vi "Boolean Array to Matlab String.vi"(8 "error in (no error)":errorcluster, 10 "Value":bool[][](array[boolean]), 11 "Variable name":string) -> (0 "error out":errorcluster, 3 "String":string)   [LabVIEW 2014, in "Matlab API.lvlib"]
uses:
  Matlab API.lvlib
panel:
  out "Array":u8[](array[numeric]) format="%x"
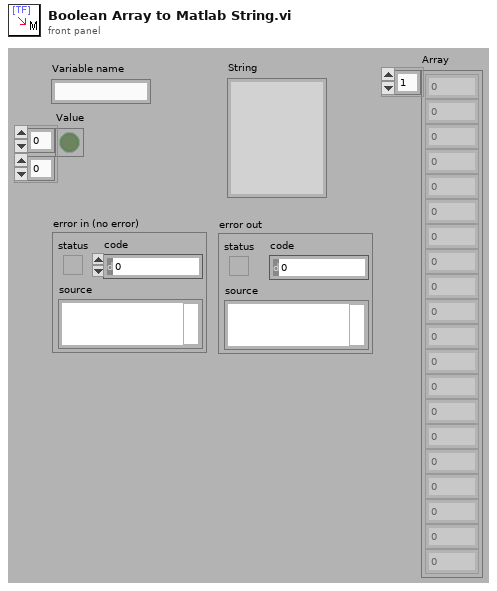
[diagram p1: front panel]
types:
  T1 = enum16{"big-endian, network order", "native, host order", "little-endian"}
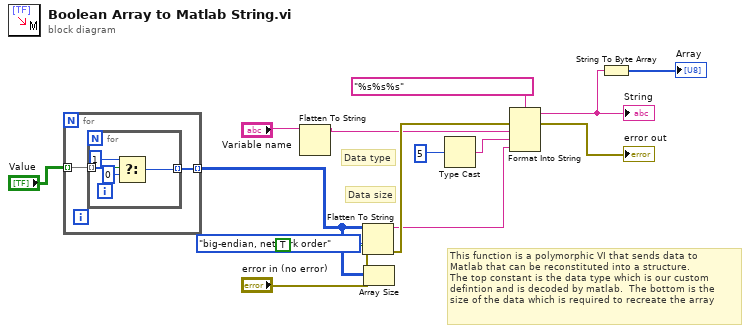
[diagram p0: block diagram]
diagram:
  # "Data size"
  # "Data type"
  # "This function is a polymorphic VI that sends data to\nMatlab that can be reconstituted into a structure.\nThe top constant is the data type which is our custom\ndefintion and is decoded by matlab.  The bottom is the\nsize of the data which is required to recreate the array"
  n1 = for {
    tunnel: "Value" -> [w17] mode=indexing
    tunnel: [w16] -> w1 mode=indexing
    n2 = for {
      tunnel: w17 -> [w21] mode=indexing
      tunnel: [w20] -> w16 mode=indexing
      n3 = Select(t=u8 1, s=w21, f=u8 0) -> (s? t:f=w20:u8)
    }
  }
  n4 = Flatten To String(anything="Variable name") -> (data string=w6:string)  [unwired: 1 in, 4 out]
  n5 = Flatten To String(anything=w1, prepend array or string size? (T)=TRUE, byte order (0:big-endian, network order)=T1."big-endian, network order", error in (no error)="error in (no error)") -> (data string=w3:string, error out=w12:errorcluster)  [unwired: 1 out]
  n6 = Array Size(array=w1) -> ()  [unwired: 1 out]
  n7 = Type Cast(x=5 ("input 2")) -> (*(type *) &x=w8:string)  [unwired: 1 out]
  n8 = Format Into String(format string="%s%s%s", error in=w12, w6, w8, w3) -> (resulting string=w9:string, error out=→"error out":errorcluster)  [unwired: 1 in]
  "String" <- w9
  n9 = String To Byte Array(string=w9) -> (unsigned byte array=→"Array":u8[])
